vi "Test Base Do Not Allow Separator in Name.vi"(8 "error in (no error)":errorcluster, 11 "Base Test in":refnum<class "Base Test.lvclass">) -> (0 "error out":errorcluster, 3 "Base Test out":refnum<class "Base Test.lvclass">)   [LabVIEW 2020, in "Base Test.lvclass"]
uses:
  Base Test.lvclass
  C:/Program Files (x86)/National Instruments/LabVIEW 2020/vi.lib/Asteme/LUnit/Test Case.lvclass
  Framework/Base/Base.lvclass
  <vilib>/Asteme/LUnit/Test Case.lvclass/Test Case.ctl
  <vilib>/Asteme/LUnit/LUnit Assertion Result.lvclass/LUnit Assertion Result.ctl
  <vilib>/Asteme/LUnit/Palette/Pass.vi
  <vilib>/Asteme/LUnit/Palette/Fail.vi
  <vilib>/Asteme/LUnit/Variant to string.vi
  <vilib>/Asteme/LUnit/Set Assertion Type.vi
  <vilib>/Asteme/LUnit/Add test result.vi
  <vilib>/Asteme/LUnit/LUnit Write Passed.vi
  <vilib>/Asteme/LUnit/LUnit Get Test Case.vi
  <vilib>/Asteme/LUnit/Assertion Result/LUnit Get Test Name.vi
  <vilib>/Asteme/LUnit/LUnit Write Message.vi
  <vilib>/Asteme/LUnit/LUnit Write Description.vi
  <vilib>/Asteme/LUnit/LUnit Write Assertion Type.vi
  <vilib>/Asteme/LUnit/Read Test Case Name.vi
  <vilib>/Utility/Data Type/Get Type Information.vi
  <vilib>/Utility/LVClass/Get LV Class Name.vi
  <vilib>/Asteme/LUnit/LUnit Assertion Result.lvclass
  <vilib>/Asteme/LUnit/Test Case.lvclass
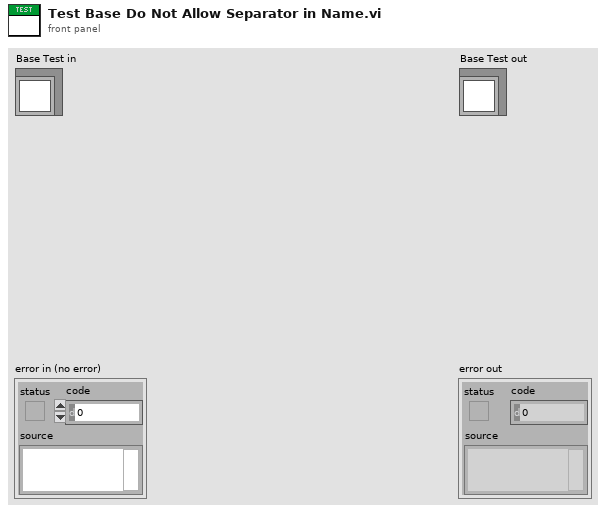
[diagram p1: front panel]
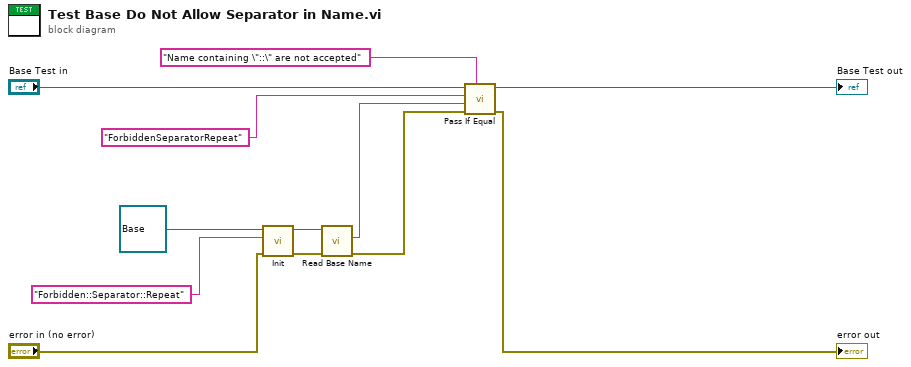
[diagram p0: block diagram]
diagram:
  n1 = call-dynamic "Init.vi"("error in (no error)"="error in (no error)", "Name"="Forbidden::Separator::Repeat", "Base In"=refnum<class "Base.lvclass"> refnum ("Base.lvclass")) -> ("error out"=w8:errorcluster, "Base Out"=w5:refnum<class "Base.lvclass">)  [unwired: 7 in]
  n2 = call-dynamic "Read Base Name.vi"("error in (no error)"=w8, "Base In"=w5) -> ("error out"=w3:errorcluster, "Name"=w1:string)  [unwired: 7 in, 1 out]
  n3 = call <vilib>:"Pass If Equal.vi"("Description"="Name containing \"::\" are not accepted", "error in (no error)"=w3, "Actual"=w1, "Expected"="ForbiddenSeparatorRepeat" ("Name"), "Test Case In"="Base Test in") -> ("error out"=→"error out":errorcluster, "Test Case Out"=→"Base Test out":refnum<class "Base Test.lvclass">)  [unwired: 5 in]
